vi "GroveFan.vi"() -> ()   [LabVIEW 2024]
uses:
  Driver/Public/Digital Direction.ctl
  Driver/CTIPicoVISA.lvlib
panel:
  out "Fan":bool
  in  "Boolean":bool
  out "Identity":T1
  in  "GroveConnector":enum16{"D16", "D18", "D20"}(ring)
  in  "stop":bool
  in  "VISA resource name in":refnum<visa-resource-name>
  out "error out":errorcluster
  # "https://wiki.seeedstudio.com/Grove-Mini_Fan/"
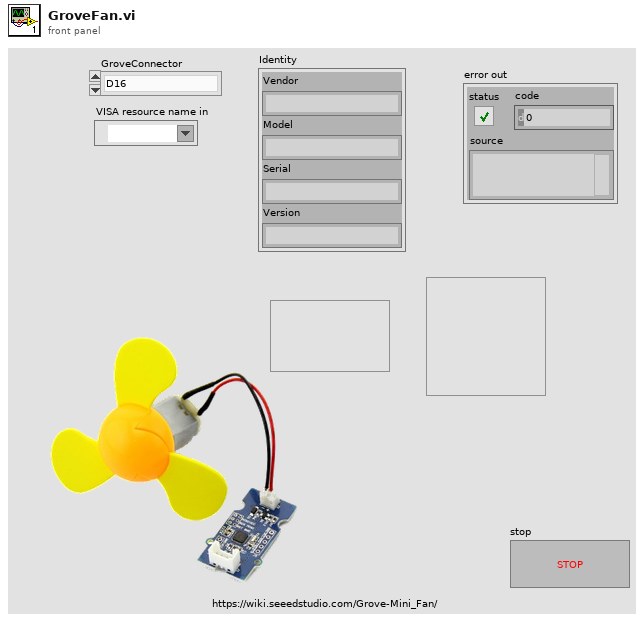
[diagram p1: front panel]
types:
  T1 = cluster{"Vendor":string, "Model":string, "Serial":string, "Version":string}
  T2 = typedef "CTIPicoVISA.lvlib/Digital Direction.ctl" = enum16{"In", "Out"}
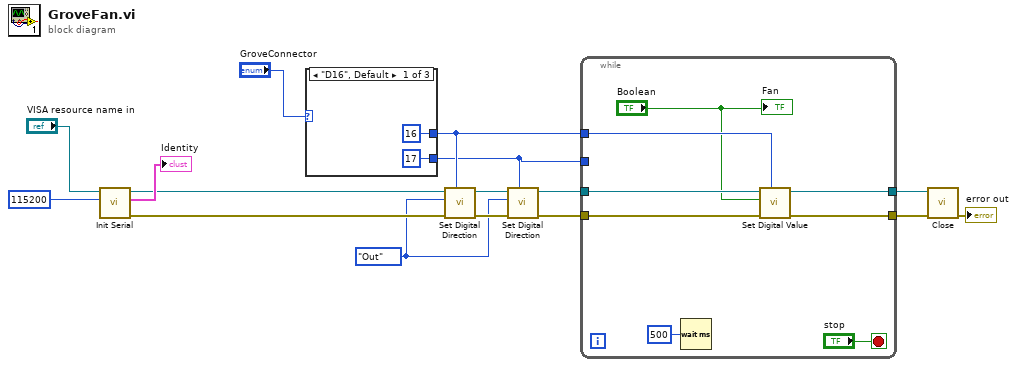
[diagram p0: block diagram]
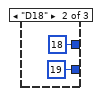
[diagram p2: hidden frame]
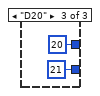
[diagram p3: hidden frame]
diagram:
  w8 = Digital_Direction."Out" ("Direction")
  n1 = call "Init Serial.vi"("Baud (115200)"=u32 115200, "VISA resource name in"="VISA resource name in") -> ("error out"=w10:errorcluster, "Identity"=→"Identity":T1, "VISA resource name Out"=w12:refnum<visa-resource-name>)  [unwired: 7 in]
  n2 = case shown="\"D16\", Default" "GroveConnector" {
    tunnel: [16 ("GPIO") 18 ("GPIO") 20 ("GPIO")] -> w11
    tunnel: [17 ("GPIO") 19 ("GPIO") 21 ("GPIO")] -> w6
    frame "D16", Default {
    }
    frame "D18" {
    }
    frame "D20" {
    }
  }
  n3 = call "Set Digital Direction.vi"("GPIO"=w11, "error in (no error)"=w10, "Direction"=w8, "VISA resource name in"=w12) -> ("error out"=w9:errorcluster, "VISA resource name"=w7:refnum<visa-resource-name>)  [unwired: 6 in]
  n4 = call "Set Digital Direction.vi"("GPIO"=w6, "error in (no error)"=w9, "Direction"=w8, "VISA resource name in"=w7) -> ("error out"=w4:errorcluster, "VISA resource name"=w5:refnum<visa-resource-name>)  [unwired: 6 in]
  n5 = while {
    tunnel: w4 -> [w27]
    tunnel: w5 -> [w28]
    tunnel: [w25] -> w3
    tunnel: [w24] -> w2
    tunnel: w11 -> [w26]
    tunnel: w6 -> [_]
    stop <- "stop" stop-if-true
    n6 = Wait (ms)(milliseconds to wait=u32 500) -> ()  [unwired: 1 out]
    n7 = call "Set Digital Value.vi"("GPIO"=w26, "error in (no error)"=w27, "Value"="Boolean", "VISA resource name in"=w28) -> ("error out"=w24:errorcluster, "VISA resource name"=w25:refnum<visa-resource-name>)  [unwired: 6 in]
    "Fan" <- "Boolean"
  }
  n8 = call "Close.vi"("error in (no error)"=w2, "VISA resource name in"=w3) -> ("error out"=→"error out":errorcluster)  [unwired: 9 in]
